vi "pair modules.vi"(5 "paired target in":refnum<class "Targets.lvclass">, 6 "paired engine in":refnum<class "engine configuration.lvclass">, 7 "target in":refnum<class "Targets.lvclass">, 8 "error in":errorcluster, 9 "engine configuration in":refnum<class "engine configuration.lvclass">, 10 "module to pair with":refnum<class "TEC editor node.lvclass">, 11 "UDP Broadcast Editor Node in":refnum<class "TEC editor node.lvclass">) -> (0 "error out":errorcluster, 1 "engine configuration out":refnum<class "engine configuration.lvclass">, 2 "module to pair with out":refnum<class "TEC editor node.lvclass">, 3 "UDP Broadcast Editor Node out":refnum<class "TEC editor node.lvclass">, 4 "paired engine out":refnum<class "engine configuration.lvclass">)   [LabVIEW 2013, in "TEC editor node.lvclass"]
uses:
  TEC editor node.lvclass
  <vilib>/NI/Module Execution Interface/Engine Configuration/engine configuration.lvclass
  <vilib>/NI/Tag Bus Data Framework/Configuration Editor/Classes/Targets/Targets.lvclass
  <vilib>/NI/Tag Bus Data Framework/Framework Configuration Classes/target configuration/PL_Target Configuration.lvclass/PL_Target Configuration.ctl
  TEC editor node.lvclass/TEC editor node.ctl
  <vilib>/NI/Configuration Framework/serializable configuration/NISE_CEF_serializable configuration.lvclass/NISE_CEF_serializable configuration.ctl
  configuration/TEC configuration.lvclass
  configuration/TEC configuration.lvclass/TEC configuration.ctl
  configuration/Read send to port.vi
  configuration/Read receive on port.vi
  configuration/Write send to address.vi
  configuration/Write receive on port.vi
  configuration/Write send to port.vi
  <vilib>/NI/Tag Bus Data Framework/Framework Configuration Classes/target configuration/Read hostname.vi
  <vilib>/NI/Tag Bus Data Framework/Configuration Editor/Classes/Targets/read target configuration.vi
  <vilib>/Utility/LVClass/Get LV Class Name.vi
  <vilib>/NI/Configuration Framework/error generator.vi
  <vilib>/NI/Configuration Framework/serializable configuration/NISE_CEF_serializable configuration.lvclass
  <vilib>/NI/Tag Bus Data Framework/Framework Configuration Classes/target configuration/PL_Target Configuration.lvclass
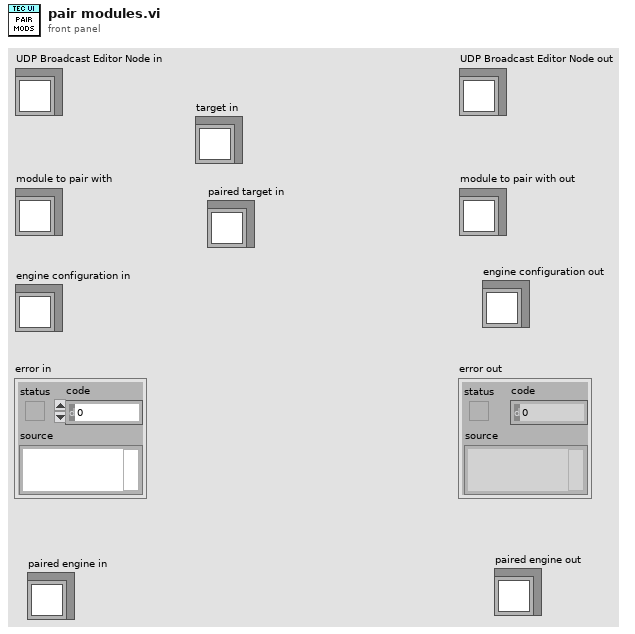
[diagram p1: front panel]
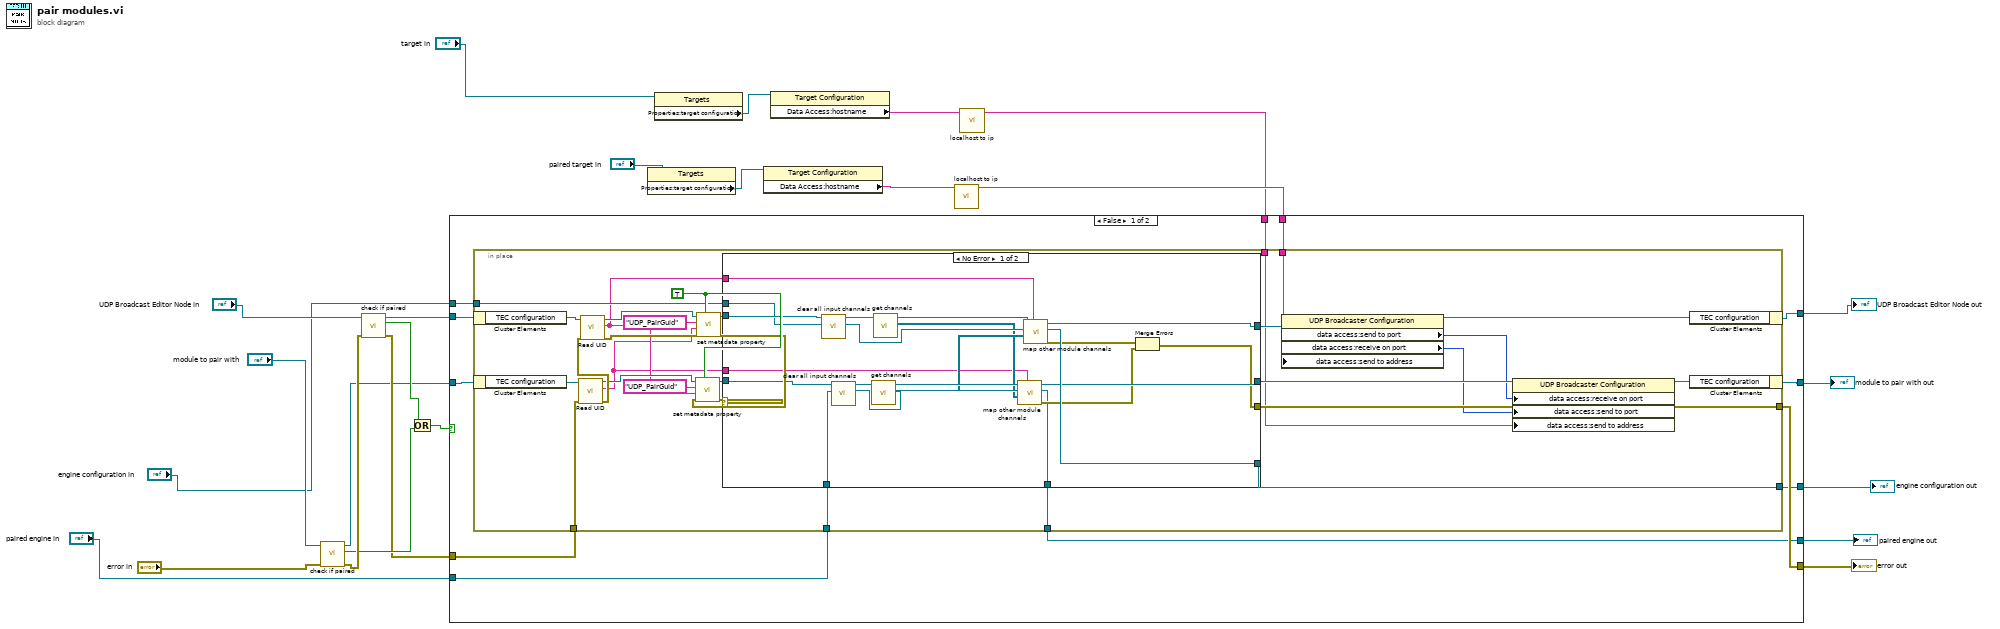
[diagram p0: block diagram]
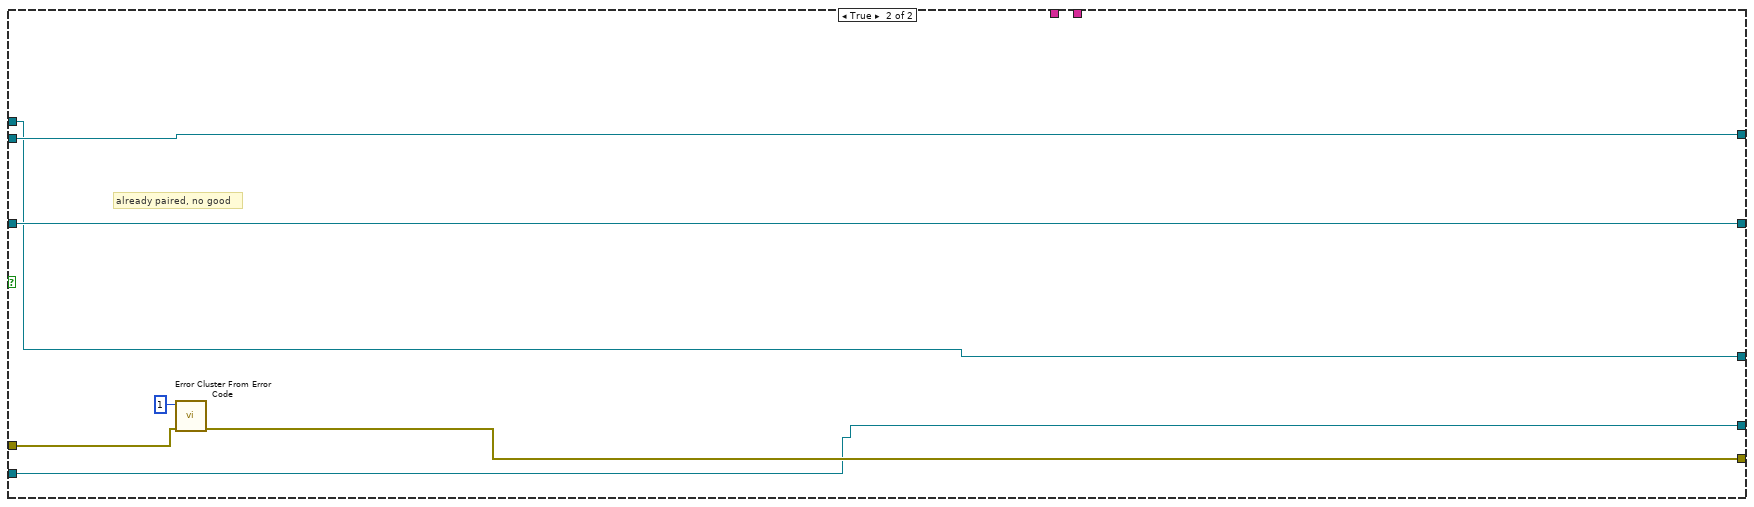
[diagram p3: hidden frame]
diagram:
  n1 = call "check if paired.vi"("error in"="error in", "UDP Broadcast Editor Node in"="module to pair with") -> ("error out"=w22:errorcluster, "paired"=w20:bool, "UDP Broadcast Editor Node out"=w14:refnum<class "TEC editor node.lvclass">)  [unwired: 7 in]
  n2 = call "check if paired.vi"("error in"=w22, "UDP Broadcast Editor Node in"="UDP Broadcast Editor Node in") -> ("error out"=w18:errorcluster, "paired"=w21:bool, "UDP Broadcast Editor Node out"=w15:refnum<class "TEC editor node.lvclass">)  [unwired: 7 in]
  n3 = Or(x=w21, y=w20) -> (x .or. y?=w19:bool)
  n4 = property class="Targets"(reference="paired target in") -> ("Properties:target configuration"=w7:refnum<class "PL_Target Configuration.lvclass">)  [unwired: 1 in, 2 out]
  n5 = property class="Targets"(reference="target in") -> ("Properties:target configuration"=w6:refnum<class "PL_Target Configuration.lvclass">)  [unwired: 1 in, 2 out]
  n6 = property class="Target Configuration"(reference=w7) -> ("Data Access:hostname"=w4:string)  [unwired: 1 in, 2 out]
  n7 = property class="Target Configuration"(reference=w6) -> ("Data Access:hostname"=w2:string)  [unwired: 1 in, 2 out]
  n8 = call "localhost to ip.vi"("hostname"=w4) -> ("true hostname"=w3:string)  [unwired: 10 in]
  n9 = call "localhost to ip.vi"("hostname"=w2) -> ("true hostname"=w1:string)  [unwired: 10 in]
  n10 = case shown="False" w19 {
    tunnel: w18 -> [w34 w99]
    tunnel: [w33 w97] -> w17
    tunnel: [w36 w96] -> w16
    tunnel: w15 -> [w37 w96]
    tunnel: w14 -> [w35 w95]
    tunnel: [w32 w95] -> w13
    tunnel: "engine configuration in" -> [w31 w94]
    tunnel: "paired engine in" -> [w30 w93]
    tunnel: [w29 w94] -> w10
    tunnel: [w28 w93] -> w9
    tunnel: w1 -> [w27 _]
    tunnel: w3 -> [w26 _]
    frame False {
      n11 = in-place {
        in-place-border: w34 -> [w64]
        in-place-border: [w54] -> w33
        in-place-border: w31 -> [w49]
        in-place-border: w30 -> [w48]
        in-place-border: [w46] -> w29
        in-place-border: [w45] -> w28
        in-place-border: w27 -> [w39]
        in-place-border: w26 -> [w38]
        w60 = TRUE ("overwrite?")
        n12 = in-place-cluster #1(w37) -> ("TEC configuration"=w66:refnum<class "TEC configuration.lvclass">)
        n13 = in-place-cluster #2(w35) -> ("TEC configuration"=w65:refnum<class "TEC configuration.lvclass">)
        n14 = call <vilib>:"Read UID.vi"("error in"=w64, "configuration in"=w65) -> ("error out"=w63:errorcluster, "instance id"=w44:string, "configuration out"=w58:refnum<class "TEC configuration.lvclass">)  [unwired: 7 in]
        n15 = call <vilib>:"Read UID.vi"("error in"=w63, "configuration in"=w66) -> ("error out"=w57:errorcluster, "instance id"=w47:string, "configuration out"=w59:refnum<class "TEC configuration.lvclass">)  [unwired: 7 in]
        n16 = call <vilib>:"set metadata property.vi"("overwrite?"=w60, "error in"=w57, "value"=w44, "key"="UDP_PairGuid", "configuration in"=w59) -> ("error out"=w56:errorcluster, "configuration out"=w50:refnum<class "TEC configuration.lvclass">)  [unwired: 5 in]
        n17 = call <vilib>:"set metadata property.vi"("overwrite?"=w60, "error in"=w56, "value"=w47, "key"="UDP_PairGuid", "configuration in"=w58) -> ("error out"=w55:errorcluster, "configuration out"=w53:refnum<class "TEC configuration.lvclass">)  [unwired: 5 in]
        n18 = case shown="No Error" w55 {
          selector: w55 -> [_ w92]
          tunnel: [w73 w92] -> w54
          tunnel: w53 -> [w87 w91]
          tunnel: [w74 w91] -> w52
          tunnel: [w79 w90] -> w51
          tunnel: w50 -> [w86 w90]
          tunnel: w49 -> [w83 w88]
          tunnel: w48 -> [w81 w89]
          tunnel: w47 -> [w76 _]
          tunnel: [w78 w88] -> w46
          tunnel: [w71 w89] -> w45
          tunnel: w44 -> [w67 _]
          frame No Error {
            n19 = call "clear all input channels.vi"("engine configuration in"=w83, "TEC configuration in"=w86) -> ("engine configuration out"=w82:refnum<class "engine configuration.lvclass">, "TEC configuration out"=w85:refnum<class "TEC configuration.lvclass">)  [unwired: 8 in]
            n20 = call "clear all input channels.vi"("engine configuration in"=w81, "TEC configuration in"=w87) -> ("engine configuration out"=w70:refnum<class "engine configuration.lvclass">, "TEC configuration out"=w84:refnum<class "TEC configuration.lvclass">)  [unwired: 8 in]
            n21 = call-dynamic "get channels.vi"("TEC configuration in"=w84) -> ("channels"=w69:refnum<class "TBM channel.lvclass">[], "TEC configuration out"=w75:refnum<class "TEC configuration.lvclass">)  [unwired: 9 in]
            n22 = call-dynamic "get channels.vi"("TEC configuration in"=w85) -> ("channels"=w68:refnum<class "TBM channel.lvclass">[], "TEC configuration out"=w80:refnum<class "TEC configuration.lvclass">)  [unwired: 9 in]
            n23 = call "map other module channels.vi"("instance id"=w67, "channels"=w68, "engine configuration in"=w70, "TEC configuration in"=w75) -> ("error out"=w72:errorcluster, "engine configuration out"=w71:refnum<class "engine configuration.lvclass">, "TEC configuration out"=w74:refnum<class "TEC configuration.lvclass">)  [unwired: 5 in]
            n24 = call "map other module channels.vi"("instance id"=w76, "channels"=w69, "engine configuration in"=w82, "TEC configuration in"=w80) -> ("error out"=w77:errorcluster, "engine configuration out"=w78:refnum<class "engine configuration.lvclass">, "TEC configuration out"=w79:refnum<class "TEC configuration.lvclass">)  [unwired: 5 in]
            n25 = Merge Errors(w77, w72) -> (w73:errorcluster)
          }
          frame Error {
          }
        }
        n26 = property class="UDP Broadcaster Configuration"(reference=w51, "data access:send to address"=w38) -> (reference out=w42:refnum<class "TEC configuration.lvclass">, "data access:send to port"=w40:u16, "data access:receive on port"=w41:u16)  [unwired: 1 in, 1 out]
        n27 = property class="UDP Broadcaster Configuration"(reference=w52, "data access:receive on port"=w40, "data access:send to port"=w41, "data access:send to address"=w39) -> (reference out=w43:refnum<class "TEC configuration.lvclass">)  [unwired: 1 in, 1 out]
        n28 = in-place-cluster #1("TEC configuration"=w42) -> (w36:refnum<class "TEC editor node.lvclass">)
        n29 = in-place-cluster #2("TEC configuration"=w43) -> (w32:refnum<class "TEC editor node.lvclass">)
      }
    }
    frame True {
      # "already paired, no good"
      n30 = call <vilib>:"Error Cluster From Error Code.vi"("error in (no error)"=w99, "error code (0)"=1) -> ("error out"=w97:errorcluster)  [unwired: 7 in]
    }
  }
  "error out" <- w17
  "UDP Broadcast Editor Node out" <- w16
  "module to pair with out" <- w13
  "engine configuration out" <- w10
  "paired engine out" <- w9
